vi "MoveStepCommand.vi"(8 "error in (no error)":errorcluster, 10 "MultiCVT":bool, 11 "Tapedrive_ESP301 in":refnum<class "Tapedrive_ESP301.lvclass">) -> (0 "error out":errorcluster, 2 "String":string, 3 "Tapedrive_ESP301.lvclass":refnum<class "Tapedrive_ESP301.lvclass">)   [LabVIEW 2011, in "Tapedrive_ESP301.lvclass"]
uses:
  Tapedrive_ESP301.lvclass
  Tapedrive_ESP301.lvclass/Tapedrive_ESP301.ctl
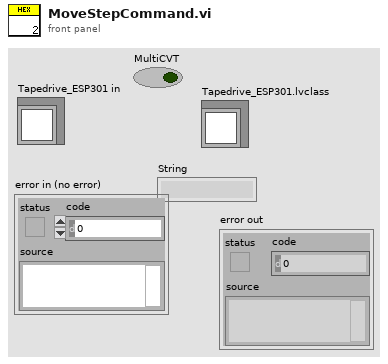
[diagram p1: front panel]
types:
  T1 = typedef "Direction.ctl" = enum16{"Forward", "Backward", "Undefined"}
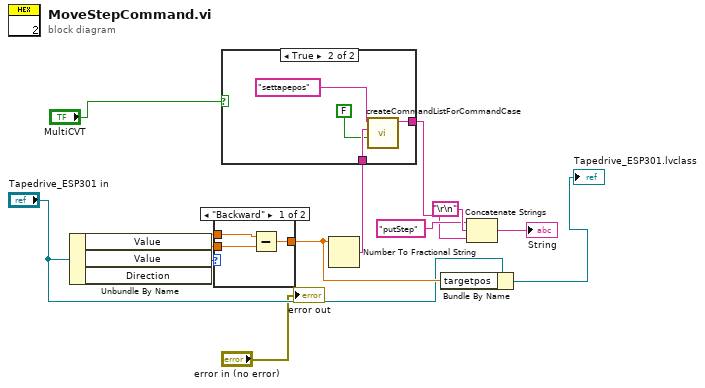
[diagram p0: block diagram]
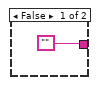
[diagram p2: hidden frame]
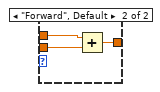
[diagram p3: hidden frame]
diagram:
  n1 = Unbundle By Name("Tapedrive_ESP301 in") -> ("Value"=w10:dbl, "Value"=w9:dbl, "Direction"=w11:T1)
  n2 = case shown="\"Backward\"" w11 {
    tunnel: w9 -> [w16 w18]
    tunnel: w10 -> [w15 w19]
    tunnel: [w14 w17] -> w12
    frame "Backward" {
      n3 = Subtract(x=w16, y=w15) -> (x-y=w14:dbl)
    }
    frame "Forward", Default {
      n4 = Add(x=w18, y=w19) -> (x+y=w17:dbl)
    }
  }
  n5 = Number To Fractional String(number=w12) -> (F-format string=w13:string)  [unwired: 3 in]
  n6 = case shown="True" "MultiCVT" {
    tunnel: w13 -> [_ w24]
    tunnel: ["" w21] -> w1
    frame False {
    }
    frame True {
      n7 = call "createCommandListForCommandCase.vi"("immediate Check (only once)"=FALSE, "setvalue"=w24, "command"="settapepos") -> ("new commands"=w21:string)  [unwired: 8 in]
    }
  }
  n8 = Bundle By Name(cluster="Tapedrive_ESP301 in", "targetpos"=w12) -> (→"Tapedrive_ESP301.lvclass":refnum<class "Tapedrive_ESP301.lvclass">)
  n9 = Concatenate Strings("putStep" ("string"), "\r\n", w1) -> (→"String":string)
  "error out" <- "error in (no error)"
